vi "HXG2_SAVE-PID_gains_gainscheduling.vi"(8 "error in":errorcluster, 11 "PID Setup Array":T2) -> (0 "error out":errorcluster)   [LabVIEW 2012]
uses:
  PID/HXG2_Horizontal PID Control.ctl
  <vilib>/Utility/file.llb/Write To Spreadsheet File (DBL).vi
panel:
  in  "LiqHeat Cascade":T1={"PID gains"={"proportional gain (Kc)"=3.54, "integral time (Ti, min)"=46.25, "derivative time (Td, min)"=0.0}, "output range"={"output high"=100.0, "output low"=0.0}} {"output range"."output low" format="%.2f"; "output range"."output high" format="%.2f"; "PID gains"."derivative time (Td, min)" format="%.3f"; "PID gains"."integral time (Ti, min)" format="%.3f"; "PID gains"."proportional gain (Kc)" format="%.3f"}
  in  "AirCool Cascade":T1={"PID gains"={"proportional gain (Kc)"=-1.15, "integral time (Ti, min)"=2.44, "derivative time (Td, min)"=0.0}, "output range"={"output high"=100.0, "output low"=10.0}} {"output range"."output low" format="%.2f"; "output range"."output high" format="%.2f"; "PID gains"."derivative time (Td, min)" format="%.3f"; "PID gains"."integral time (Ti, min)" format="%.3f"; "PID gains"."proportional gain (Kc)" format="%.3f"}
  out "size(s)":i32
  out "appended array":dbl[](array[numeric])
  out "To File":dbl[][](array[numeric])
  out "deleted path":path
  # "P"
  # "I"
  # "D"
  # "Max PV"
  # "UL"
  # "LL"
  # "Three rows per system"
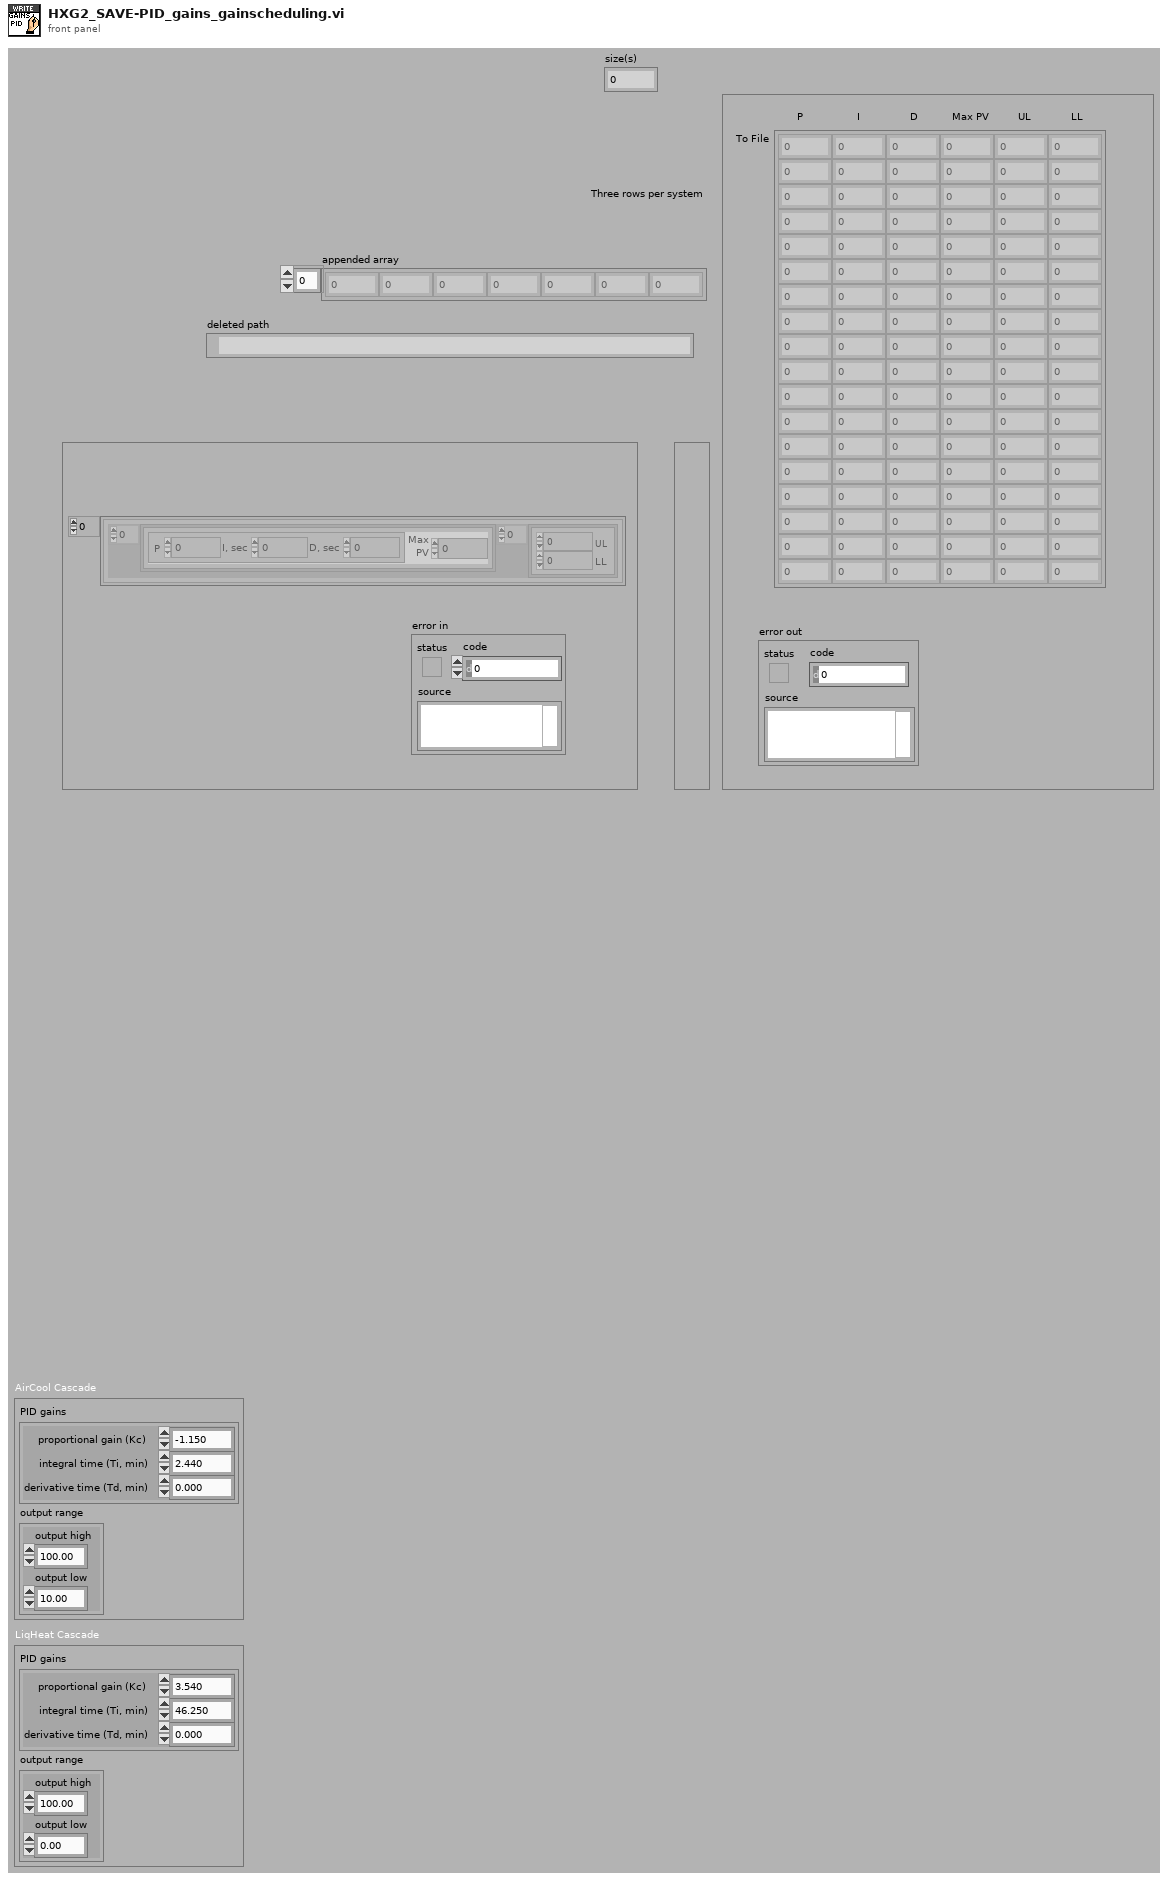
[diagram p1: front panel]
types:
  T1 = cluster{"PID gains":cluster{"proportional gain (Kc)":dbl, "integral time (Ti, min)":dbl, "derivative time (Td, min)":dbl}, "output range":cluster{"output high":dbl, "output low":dbl}}
  T2 = typedef "HXG2_Horizontal PID Control.ctl" = cluster{"GainsArray":cluster{"Gains 2":cluster{"P":dbl, "I, sec":dbl, "D, sec":dbl}, "Max\nPV":dbl}[], "UL-LL Array":cluster{"UL":dbl, "LL  ":dbl}[]}[]
  T3 = cluster{"Gains 2":cluster{"P":dbl, "I, sec":dbl, "D, sec":dbl}, "Max\nPV":dbl}[]
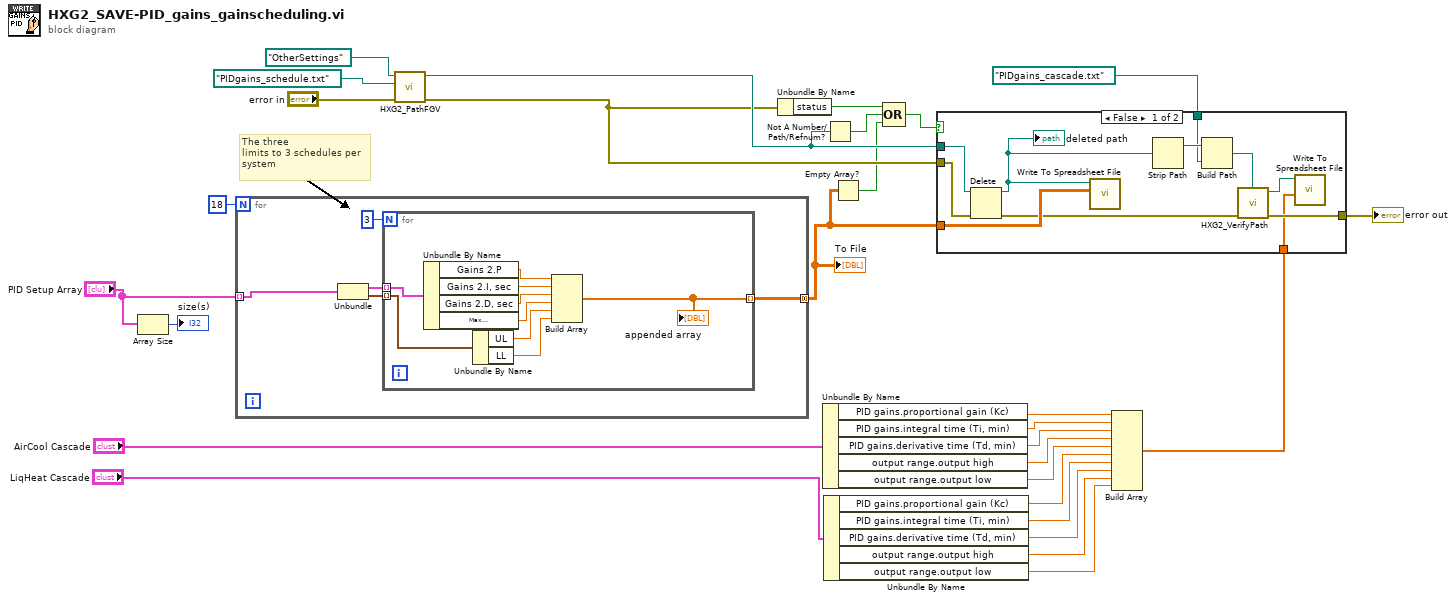
[diagram p0: block diagram]
diagram:
  # "The three\nlimits to 3 schedules per\nsystem"
  n1 = Array Size(array="PID Setup Array") -> (size(s)=→"size(s)":i32)
  n2 = for {
    N: 18 -> [_]
    tunnel: "PID Setup Array" -> [w33] mode=indexing
    tunnel: [w30] -> w17 mode=concatenating
    n3 = Unbundle(w33) -> ("GainsArray"=w32:T3, "UL-LL Array"=w31:cluster{"UL":dbl, "LL  ":dbl}[])
    n4 = for {
      N: 3 -> [_]
      tunnel: w32 -> [w36] mode=indexing
      tunnel: w31 -> [w35] mode=indexing
      tunnel: [w34] -> w30 mode=indexing
      n5 = Unbundle By Name(w36) -> ("Gains 2.P"=w42:dbl, "Gains 2.I, sec"=w41:dbl, "Gains 2.D, sec"=w40:dbl, "Max\nPV"=w39:dbl)
      n6 = Unbundle By Name(w35) -> ("UL"=w38:dbl, "LL"=w37:dbl)
      n7 = Build Array(w42, w41, w40, w39, w38, w37) -> (w34:dbl[])
      "appended array" <- w34
    }
  }
  "To File" <- w17
  n8 = call "HXG2_PathFGV.vi"("error in (no error)"="error in", "File Name"=path "PIDgains_schedule.txt", "Folder Name"=path "OtherSettings") -> ("error out"=w21:errorcluster, "File path"=w22:path)  [unwired: 5 in, 2 out]
  n9 = Unbundle By Name(w21) -> ("status"=w25:bool)
  n10 = Unbundle By Name("AirCool Cascade") -> ("PID gains.proportional gain (Kc)"=w11:dbl, "PID gains.integral time (Ti, min)"=w10:dbl, "PID gains.derivative time (Td, min)"=w9:dbl, "output range.output high"=w8:dbl, "output range.output low"=w7:dbl)
  n11 = Unbundle By Name("LiqHeat Cascade") -> ("PID gains.proportional gain (Kc)"=w6:dbl, "PID gains.integral time (Ti, min)"=w5:dbl, "PID gains.derivative time (Td, min)"=w4:dbl, "output range.output high"=w3:dbl, "output range.output low"=w2:dbl)
  n12 = Not A Number/Path/Refnum?(number/path/refnum=w22) -> (NaN/Path/Refnum?=w26:bool)
  n13 = Empty Array?(array=w17) -> (empty?=w19:bool)
  n14 = Compound Arithmetic op=OR(w25, w26, w19) -> (w28:bool)
  n15 = Build Array(w11, w10, w9, w8, w7, w6, w5, w4, w3, w2) -> (w1:dbl[])
  n16 = case shown="False" w28 {
    tunnel: w17 -> [w51 _]
    tunnel: w22 -> [w53 _]
    tunnel: w21 -> [w52 w54]
    tunnel: [w45 w54] -> w27
    tunnel: path "PIDgains_cascade.txt" -> [w48 _]
    tunnel: w1 -> [w43 _]
    frame False {
      n17 = Delete(path (use dialog)=w53, error in=w52) -> (deleted path=w50:path, error out=w46:errorcluster)  [unwired: 4 out]
      "deleted path" <- w50
      n18 = call-poly <vilib>:"Write To Spreadsheet File.vi"("2D data"=w51, "file path (dialog if empty)"=w50) -> ()  [unwired: 4 in, 3 out]
      n19 = Strip Path(path=w50) -> (stripped path=w49:path)  [unwired: 1 out]
      n20 = Build Path(base path=w49, name or relative path=w48) -> (appended path=w47:path)
      n21 = call "HXG2_VerifyPath.vi"("error in (no error)"=w46, "Path In"=w47) -> ("error out"=w45:errorcluster, "Path Out"=w44:path)  [unwired: 8 in]
      n22 = call-poly <vilib>:"Write To Spreadsheet File.vi"("1D data"=w43, "file path (dialog if empty)"=w44) -> ()  [unwired: 4 in, 3 out]
    }
    frame True {
    }
  }
  "error out" <- w27
